vi "Publisher-right.vi"() -> ()   [LabVIEW 2014]
uses:
  <vilib>/Tufts CEEO ROS for LabVIEW Software/ROS/Code/Console/Servers/ServerSubs/TopicDef.ctl
  <vilib>/Tufts CEEO ROS for LabVIEW Software/ROS/Code/SubVIs/_ROSDirection.ctl
  ctl/pose.ctl
  ctl/Point.ctl
  ctl/RPY.ctl
panel:
  out "what I sent msg out":string
  out "Quaternion":cluster{"x":dbl, "y":dbl, "z":dbl, "w":dbl}
  out "error out":errorcluster
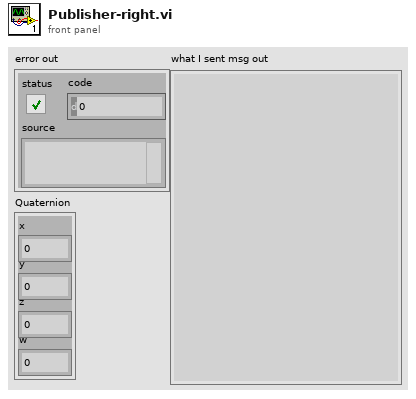
[diagram p1: front panel]
types:
  T1 = typedef "TopicDef.ctl" = cluster{"Topic":string, "Type":string, "Action":T2, "Update (ms)":u16, "queue size":u16}
  T2 = typedef "_ROSDirection.ctl" = enum16{"Node", "Publisher", "Subscriber", "ServiceClient", "ServiceProvider"}
  T3 = typedef "_ROSControl.ctl" = cluster{"topic port":u16, "Node":string, "topic":string, "type":string, "node port":u16, "error ":errorcluster, "Direction":T2, "Update (ms)":u16, "FIFO size":u16}
  T4 = typedef "RPY.ctl" = cluster{"Roll (y)":dbl, "Pitch (x)":dbl, "Yaw (z)":dbl}
  T5 = typedef "Point.ctl" = cluster{"x":dbl, "y":dbl, "z":dbl}
  T6 = typedef "pose.ctl" = cluster{"Point":cluster{"x":dbl, "y":dbl, "z":dbl}, "Quaternion":cluster{"x":dbl, "y":dbl, "z":dbl, "w":dbl}}
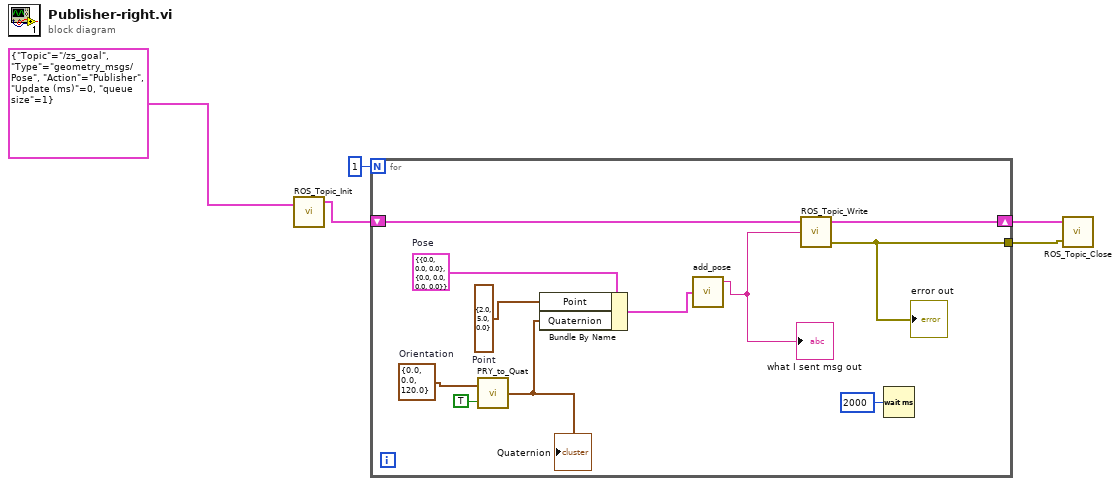
[diagram p0: block diagram]
diagram:
  n1 = call <vilib>:"ROS_Topic_Init.vi"("Definitions"=T1 {"Topic"="/zs_goal", "Type"="geometry_msgs/Pose", "Action"=enum."Publisher", "Update (ms)"=0, "queue size"=1}) -> ("ROS out"=w2:T3)  [unwired: 2 in, 1 out]
  n2 = for {
    N: 1 -> [_]
    tunnel: [w16] -> w5
    shift-right: [w15] -> w4
    shift-left: w2 -> [w14]
    w12 = T4 {"Roll (y)"=0.0, "Pitch (x)"=0.0, "Yaw (z)"=120.0}  # Orientation
    w10 = T5 {"x"=2.0, "y"=5.0, "z"=0.0}  # Point
    w11 = T6 {"Point"={"x"=0.0, "y"=0.0, "z"=0.0}, "Quaternion"={"x"=0.0, "y"=0.0, "z"=0.0, "w"=0.0}}  # Pose
    n3 = call <vilib>:"PRY_to_Quat.vi"("From Degrees? (T)"=TRUE, "Orientation"=w12) -> ("Quaternion"=w9:cluster{"x":dbl, "y":dbl, "z":dbl, "w":dbl})
    "Quaternion" <- w9
    n4 = Bundle By Name(cluster=w11, "Point"=w10, "Quaternion"=w9) -> (w7:T6)
    n5 = call <vilib>:"add_pose.vi"("Pose"=w7) -> ("msg out"=w8:string)  [unwired: 4 in]
    "what I sent msg out" <- w8
    n6 = call <vilib>:"ROS_Topic_Write.vi"("Msg in"=w8, "ROS in"=w14) -> ("error out"=w16:errorcluster, "ROS out"=w15:T3)  [unwired: 2 in]
    "error out" <- w16
    n7 = Wait (ms)(milliseconds to wait=u32 2000 ("等待时间（毫秒）")) -> ()  [unwired: 1 out]
  }
  n8 = call <vilib>:"ROS_Topic_Close.vi"("error in"=w5, "ROS in"=w4) -> ()  [unwired: 2 in, 1 out]
